vi "Check if Create Controls Enabled.vi"() -> (3 "Create Controls/Constants Enabled?":bool)   [LabVIEW 2016, in "PantherLAB_Scripting.lvlib"]
uses:
  PantherLAB_Scripting.lvlib
  <resource>/dialog/lvconfig.llb/LV Config Read Boolean.vi
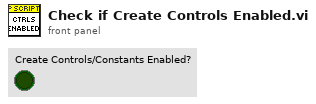
[diagram p1: front panel]
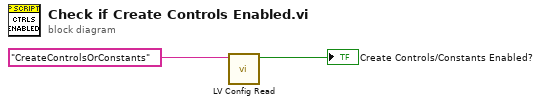
[diagram p0: block diagram]
diagram:
  n1 = call-poly <resource>:"LV Config Read.vi"("key"="CreateControlsOrConstants") -> ("value"=→"Create Controls/Constants Enabled?":bool)  [unwired: 4 in, 2 out]
